vi "GPIO Write Value.vi"(7 "GPIO #":T1=-1, 8 "error in (no error)":errorcluster, 10 "Value":bool, 11 "FirmwareComms in":refnum<class "VisaComms.lvclass">) -> (0 "error out":errorcluster, 3 "FirmwareComms out":refnum<class "VisaComms.lvclass">)   [LabVIEW 2020, in "CTI.lvlib" / "VisaComms.lvclass"]
uses:
  VisaComms.lvclass
  VisaComms.lvclass/VisaComms.ctl
  GPIO Number.ctl
  CTI.lvlib
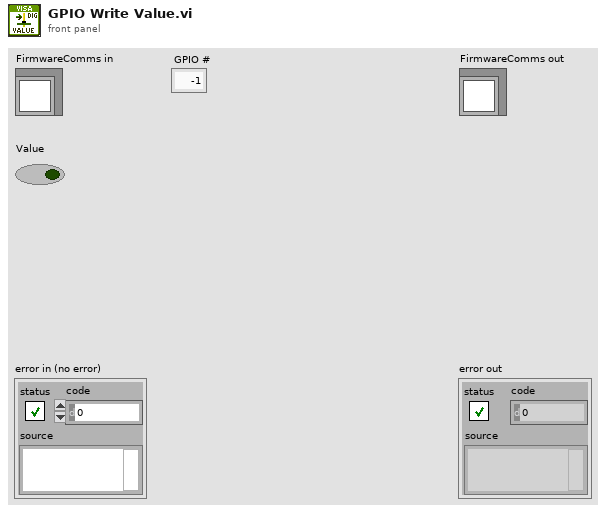
[diagram p1: front panel]
types:
  T1 = typedef "CTI.lvlib/GPIO Number.ctl" = i8
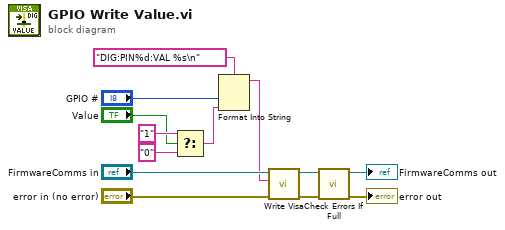
[diagram p0: block diagram]
diagram:
  n1 = Select(t="1", s="Value", f="0") -> (s? t:f=w9:string)
  n2 = Format Into String(format string="DIG:PIN%d:VAL %s\n", "GPIO #", w9) -> (resulting string=w4:string)  [unwired: 2 in, 1 out]
  n3 = call "Write Visa.vi"("error in (no error)"="error in (no error)", "write buffer"=w4, "VisaComms in"="FirmwareComms in") -> ("error out"=w2:errorcluster, "VisaComms out"=w6:refnum<class "VisaComms.lvclass">)  [unwired: 6 in, 1 out]
  n4 = call "Check Errors If Full.vi"("error in (no error)"=w2, "VisaComms in"=w6) -> ("error out"=→"error out":errorcluster, "VisaComms out"=→"FirmwareComms out":refnum<class "VisaComms.lvclass">)  [unwired: 8 in]
